vi "Open Bus Monitor.vi"(8 "error in (no error)":errorcluster, 11 "Mediator in":refnum<class "BusMediator.lvclass">) -> (0 "error out":errorcluster, 3 "Mediator out":refnum<class "BusMediator.lvclass">)   [LabVIEW 2017, in "BusMediator.lvclass"]
uses:
  BusMediator.lvclass
  <vilib>/Composed/GPM Packages/mva-framework/Source/Framework/IViewable/IViewable Messages/Open Front Panel Msg/Open Front Panel Msg.lvclass
  <vilib>/Composed/GPM Packages/mva-framework/Source/Framework/IViewable/IViewable/View Position Enum.ctl
  <vilib>/Composed/GPM Packages/mva-framework/Source/Framework/IViewable/IViewable/IViewable.lvclass
  <vilib>/ActorFramework/Message Enqueuer/Message Enqueuer.lvclass
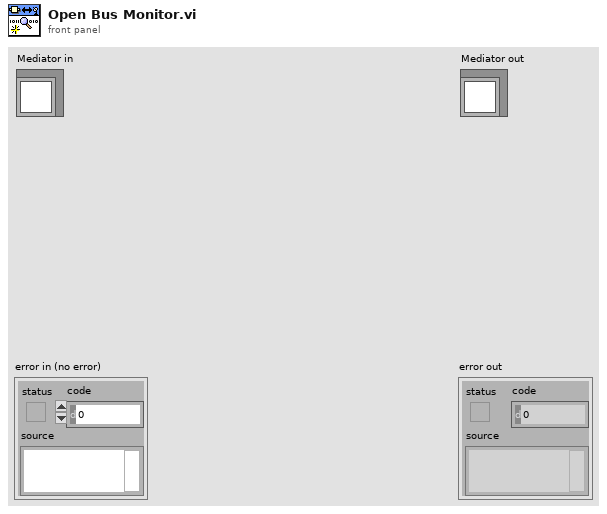
[diagram p1: front panel]
types:
  T1 = typedef "IViewable.lvlib/IViewable.lvclass/View Position Enum.ctl" = enum16{"Centered", "Maximized", "Minimized", "Custom", "Unchanged"}
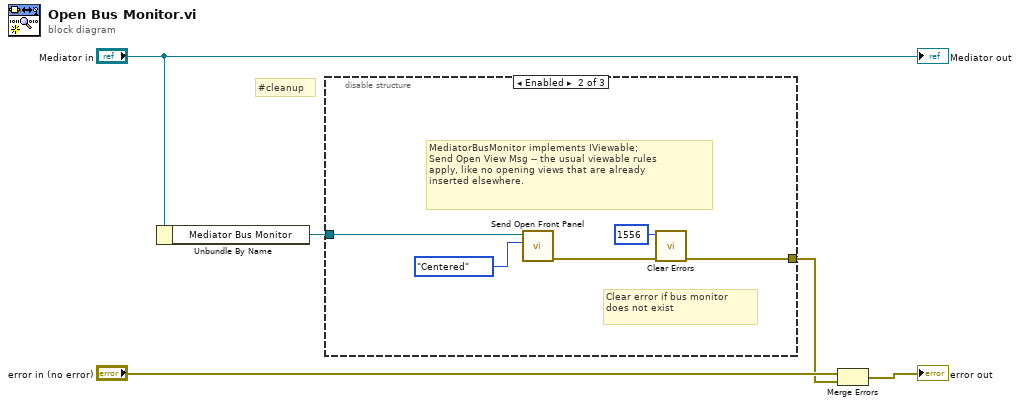
[diagram p0: block diagram]
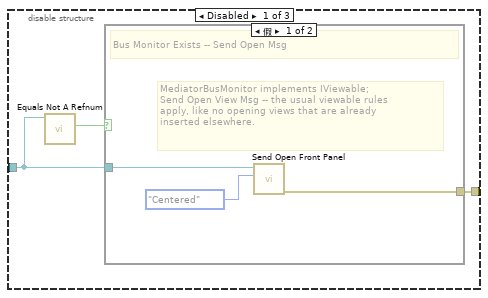
[diagram p2: hidden frame]
diagram:
  # "#cleanup"
  n1 = Unbundle By Name("Mediator in") -> ("Mediator Bus Monitor"=w1:refnum<class "Message Enqueuer.lvclass">)
  n2 = disable-structure shown="Enabled" {
    disable-tunnel: [w8 w13 _] -> w2
    disable-tunnel: w1 -> [w7 w15 _]
    frame Disabled {
      n3 = call <vilib>:"Equals Not A Refnum.vi"("Message Enqueuer"=w7) -> ("Not a refnum?"=w6:bool)  [unwired: 10 in]
      n4 = case shown="假" w6 {
        tunnel: w7 -> [w11 _]
        tunnel: [w10 _] -> w8
        frame False {
          # "MediatorBusMonitor implements IViewable;\nSend Open View Msg -- the usual viewable rules\napply, like no opening views that are already\ninserted elsewhere."
          # "Bus Monitor Exists -- Send Open Msg"
          n5 = call <vilib>:"Send Open Front Panel.vi"("Position"=View_Position_Enum."Centered", "Message Enqueuer"=w11) -> ("error out"=w10:errorcluster)  [unwired: 8 in, 1 out]
        }
        frame True {
          # "No Bus Monitor -- Send nothing"
        }
      }
    }
    frame Enabled {
      # "Clear error if bus monitor\ndoes not exist"
      # "MediatorBusMonitor implements IViewable;\nSend Open View Msg -- the usual viewable rules\napply, like no opening views that are already\ninserted elsewhere."
      n6 = call <vilib>:"Send Open Front Panel.vi"("Position"=View_Position_Enum."Centered", "Message Enqueuer"=w15) -> ("error out"=w16:errorcluster)  [unwired: 8 in, 1 out]
      n7 = call <vilib>:"Clear Errors.vi"("error in (no error)"=w16, "specific error code to clear (0: all)"=1556) -> ("error out"=w13:errorcluster)  [unwired: 4 in, 1 out]
    }
    frame Disabled {
    }
  }
  n8 = Merge Errors("error in (no error)", w2) -> (→"error out":errorcluster)
  "Mediator out" <- "Mediator in"
